vi "Main.vi"() -> ()   [LabVIEW 2016]
uses:
  type defs/action buttons.ctl
  type defs/mode buttons.ctl
  type defs/state.ctl
  type defs/data.ctl
  <vilib>/vision/Image Controls.llb/IMAQ Image.ctl
  <vilib>/myRIO/Instrument Drivers/Onboard IO/PWM/typedefs/PWM Reference.ctl
  <vilib>/myRIO/Common/Instrument Driver Framework/Utilities/typedefs/myRIO Generic Hardware Reference.ctl
  <vilib>/myRIO/Common/Instrument Driver Framework/Utilities/typedefs/Hardware Version Enum.ctl
  <vilib>/myRIO/Common/Instrument Driver Framework/Utilities/typedefs/myRIO v1.0 Reference.ctl
  <vilib>/myRIO/Common/Instrument Driver Framework/Utilities/typedefs/Generic FPGA Reference.ctl
  <vilib>/myRIO/Common/Instrument Driver Framework/myRIO v1.0/PWM/typedefs/PWM Channels Enum.ctl
  <vilib>/myRIO/Instrument Drivers/Onboard IO/PWM/typedefs/PWM Configuration.ctl
  <vilib>/userdefined/High Color/nirio_resource_hc.ctl
  <vilib>/myRIO/Instrument Drivers/Onboard IO/DIO/typedefs/DIO Reference.ctl
  <vilib>/myRIO/Common/Instrument Driver Framework/myRIO v1.0/DIO/typedefs/DIO Channels List.ctl
  <vilib>/myRIO/Common/Instrument Driver Framework/myRIO v1.0/DIO/typedefs/DIO Channels Enum.ctl
  <vilib>/myRIO/Common/Instrument Driver Framework/myRIO v1.0/Encoder/typedefs/Encoder Signal Mode.ctl
  <vilib>/myRIO/Instrument Drivers/Onboard IO/Encoder/typedefs/Encoder Reference.ctl
  <vilib>/myRIO/Common/Instrument Driver Framework/myRIO v1.0/Encoder/typedefs/Encoder Channels Enum.ctl
  <vilib>/myRIO/Common/Instrument Driver Framework/myRIO v1.0/Encoder/typedefs/Encoder Configuration v1.0.ctl
  type defs/task.ctl
  <vilib>/myRIO/Common/Instrument Driver Framework/Utilities/vis/Is FPGA Ref Available.vi
  <vilib>/myRIO/Common/Instrument Driver Framework/myRIO v1.0/PWM/vis/myRIO v1.1 Open PWM.vi
  <vilib>/myRIO/Instrument Drivers/Onboard IO/PWM/vis/Set Duty Cycle and Frequency.vi
  <vilib>/myRIO/Common/Instrument Driver Framework/myRIO v1.0/DIO/vis/myRIO v1.1 Open DIO.vi
  <vilib>/myRIO/Instrument Drivers/Onboard IO/DIO/vis/Write.vi
  <vilib>/myRIO/Common/Instrument Driver Framework/myRIO v1.0/Encoder/vis/myRIO v1.1 Open Encoder.vi
  <vilib>/myRIO/Instrument Drivers/Onboard IO/Encoder/vis/Read.vi
  <vilib>/myRIO/Instrument Drivers/Onboard IO/DIO/vis/Read.vi
  <vilib>/myRIO/Common/Instrument Driver Framework/Utilities/vis/Validate Channels.vi
  <vilib>/myRIO/Common/Instrument Driver Framework/myRIO v1.0/PWM/vis/myRIO v1.0 Reserve PWM.vi
  <vilib>/myRIO/Common/Instrument Driver Framework/myRIO v1.0/DIO/vis/myRIO v1.0 Reserve DIO.vi
  <vilib>/myRIO/Common/Instrument Driver Framework/myRIO v1.0/Encoder/vis/myRIO v1.0 Reserve Encoder.vi
  <vilib>/myRIO/Common/Instrument Driver Framework/myRIO v1.0/PWM/vis/myRIO v1.0 Build MUX Configuration PWM.vi
  <vilib>/myRIO/Common/Instrument Driver Framework/myRIO v1.0/Resource Manager/vis/myRIO v1.0 Reserve Channel List.vi
  <vilib>/myRIO/Common/Instrument Driver Framework/myRIO v1.0/DIO/vis/myRIO v1.0 Build MUX Configuration DIO.vi
  <vilib>/myRIO/Common/Instrument Driver Framework/myRIO v1.0/Encoder/vis/myRIO v1.0 Build MUX Configuration Encoder.vi
  <vilib>/myRIO/Common/Instrument Driver Framework/myRIO v1.0/Resource Manager/vis/myRIO v1.0 Create Configuration List.vi
  <vilib>/myRIO/Common/Instrument Driver Framework/myRIO v1.0/Resource Manager/vis/myRIO v1.0 Reserve Channel.vi
  <vilib>/myRIO/Common/Instrument Driver Framework/myRIO v1.0/Resource Manager/vis/myRIO v1.0 Unreserve Channel.vi
  <vilib>/myRIO/Common/Instrument Driver Framework/myRIO v1.0/Resource Manager/vis/myRIO v1.0 Build Mutex Name.vi
  <vilib>/Utility/VariantDataType/GetNumericInfo.vi
  <vilib>/Utility/error.llb/Error Cluster From Error Code.vi
  <vilib>/myRIO/Common/Instrument Driver Framework/myRIO v1.0/myRIO v1.1 Open.vi
  <vilib>/myRIO/Common/Instrument Driver Framework/Utilities/vis/IO Manager.vi
  <vilib>/myRIO/Common/Instrument Driver Framework/Utilities/vis/Configuration Manager.vi
  <vilib>/myRIO/Common/Instrument Driver Framework/myRIO v1.0/Resource Manager/vis/myRIO v1.0 Configure IO.vi
  <vilib>/myRIO/Common/Instrument Driver Framework/myRIO v1.0/myRIO v1.0 Close.vi
  <vilib>/myRIO/Common/Instrument Driver Framework/myRIO v1.0/PWM/vis/myRIO v1.0 Write PWM.vi
  <vilib>/myRIO/Common/Instrument Driver Framework/myRIO v1.0/DIO/vis/myRIO v1.0 Write DIO.vi
  <vilib>/myRIO/Common/Instrument Driver Framework/myRIO v1.0/Encoder/vis/myRIO v1.0 Configure Encoder.vi
  <vilib>/myRIO/Common/Instrument Driver Framework/myRIO v1.0/Encoder/vis/myRIO v1.0 Read Encoder.vi
  <vilib>/myRIO/Common/Instrument Driver Framework/myRIO v1.0/DIO/vis/myRIO v1.0 Read DIO.vi
  <vilib>/myRIO/Express VI/Onboard IO/PWM/PWM Express VI.xnode
  <vilib>/myRIO/Instrument Drivers/Onboard IO/PWM/vis/myRIO PWM Open.xnode
  <vilib>/myRIO/Express VI/Onboard IO/DO/DO Express VI.xnode
  <vilib>/myRIO/Instrument Drivers/Onboard IO/DIO/vis/myRIO DIO Open.xnode
  <vilib>/myRIO/Express VI/Onboard IO/Encoder/Encoder Express VI.xnode
  <vilib>/myRIO/Instrument Drivers/Onboard IO/Encoder/vis/myRIO Encoder Open.xnode
  <vilib>/myRIO/Common/Instrument Driver Framework/myRIO v1.0/Encoder/typedefs/Encoder Count Direction Enum.ctl
  <vilib>/myRIO/Express VI/Onboard Devices/LED/LED Express VI.xnode
  <vilib>/myRIO/Express VI/Onboard Devices/Button/Button Express VI.xnode
  <vilib>/vision/NI_Vision_Development_Module.lvlib
  <vilib>/myRIO/Instrument Drivers/Onboard IO/DIO/DIO.lvlib
  <vilib>/myRIO/Instrument Drivers/Onboard IO/PWM/PWM.lvlib
  <vilib>/myRIO/Instrument Drivers/Onboard IO/Encoder/Encoder.lvlib
panel:
  out "Pattern matches ball":bool
  out "Num of Matches (Color Pattern Matching 1)":i32
  out "Classes (Color Classification 1)":string[](array[string])
  out "Number of Matches (Pattern Matching 1)":i32
  out "Class (Particle Classification 1)":string
  out "Stopped":bool
  out "error out":errorcluster
  out "Boolean 2":bool
  in  "PWM 1":dbl(slide)=0.5 scale=0.0..1.0
  in  "PWM 2":dbl(slide)=0.5 scale=0.0..1.0
  out "take":bool
  in  "to give":bool
  out "Counter Value":i32
  out "Reset Counter":bool
  in  "Enum":enum16{"null", "one", "two", "stop"}(ring)=enum."two"
  out "back":bool
  out "number img":i32
  in  "mode buttons":T1
  out "image display":T2(plugin-control)
  in  "action buttons":T3
  in  "Stop":bool
  # "Machine\nVision\nApp"
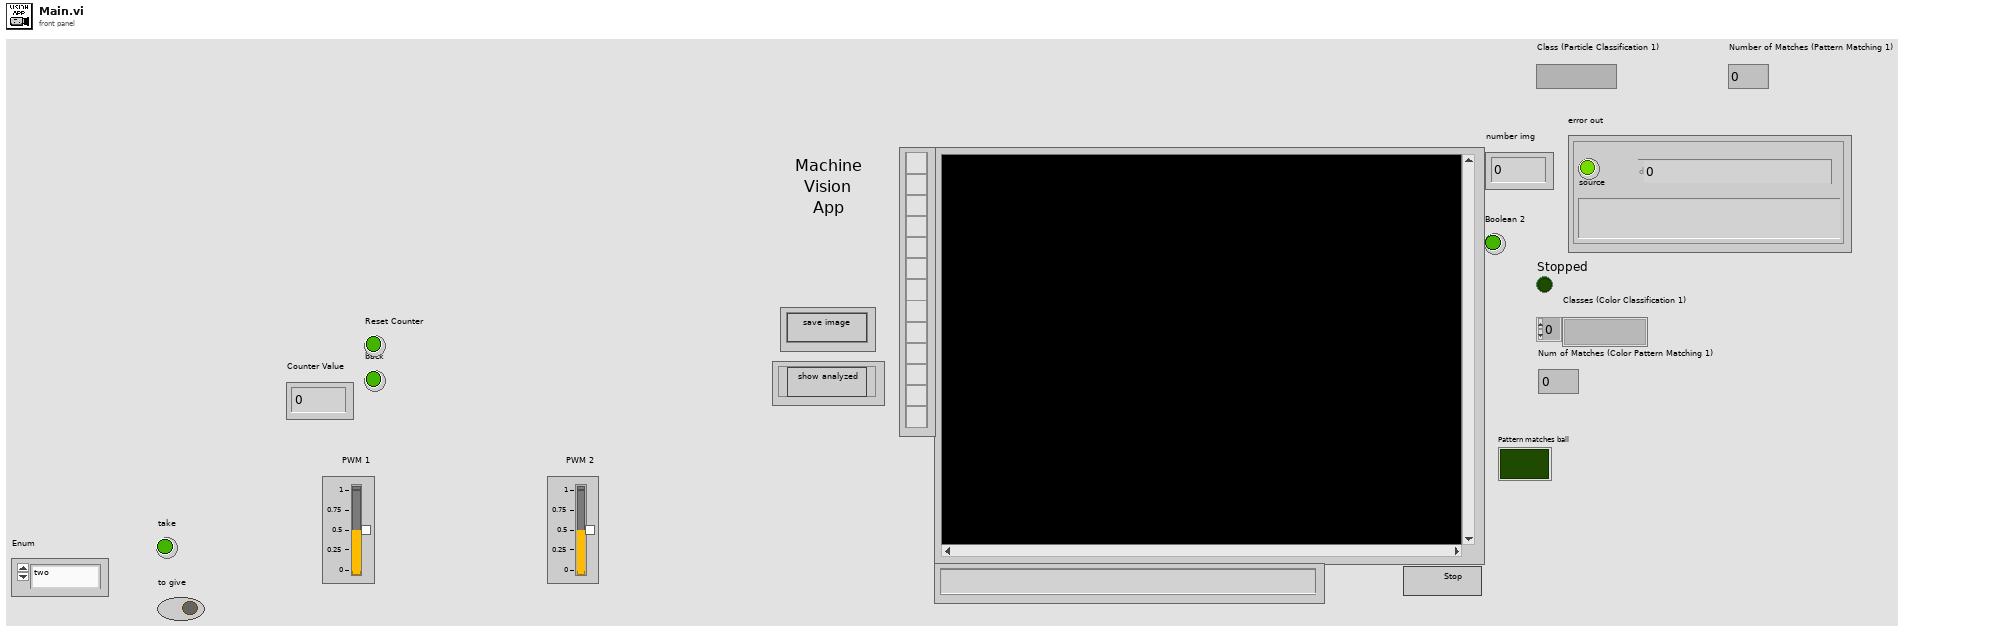
[diagram p1: front panel]
types:
  T1 = typedef "mode buttons.ctl" = cluster{"show analyzed":bool}
  T2 = typedef "IMAQ Image.ctl" = refnum<image>
  T3 = typedef "action buttons.ctl" = cluster{"save image":bool}
  T4 = typedef "data.ctl" = cluster{"save image":bool, "qsm":cluster{"Webcam image ref":T2, "Analyzed image ref":T2, "Stop webcam":bool}, " image ref":T2, "number img":i32}
  T5 = typedef "state.ctl" = enum16{"(qsm) schedule", "(qsm) initialize", "(qsm) release", "(qsm) clean up", "(qsm) shutdown", "(myRIO) initialize", "(myRIO) clean up", "(myRIO) update ports", "(image) get", "(image) analyze", "(image) overlay", "(image) show", "save image", "state A", "state B", "state C", "state D", "state E", "state F", "state G", "state H"}
  T6 = typedef "PWM.lvlib/PWM Reference.ctl" = cluster{"myRIO Reference":T7, "PWM Channels Enum":T11, "PWM Configuration":T12}
  T7 = typedef "myRIO Generic Hardware Reference.ctl" = cluster{"myRIO Model":T8, "myRIO Hardware Reference":T9}
  T8 = typedef "Hardware Version Enum.ctl" = enum16{"Unknown", "myRIO-1900", "myRIO-1950", "roboRIO", "NI ELVIS RIO CM"}
  T9 = typedef "myRIO v1.0 Reference.ctl" = cluster{"Generic FPGA Reference":T10, "Allow multiple opens":bool}
  T10 = typedef "Generic FPGA Reference.ctl" = refnum<k20>
  T11 = typedef "PWM Channels Enum.ctl" = enum16{"Not Connected", "C/PWM0", "C/PWM1", "A/PWM0", "A/PWM1", "A/PWM2", "B/PWM0", "B/PWM1", "B/PWM2", "PWM/PWM0", "PWM/PWM1", "PWM/PWM2", "PWM/PWM3", "PWM/PWM4", "PWM/PWM5", "PWM/PWM6", "PWM/PWM7", "PWM/PWM8", "PWM/PWM9"}
  T12 = typedef "PWM.lvlib/PWM Configuration.ctl" = cluster{"Frequency":dbl, "Duty Cycle":dbl}
  T13 = typedef "nirio_resource_hc.ctl" = tag
  T14 = typedef "Encoder.lvlib/Encoder Reference.ctl" = cluster{"myRIO Reference":T7, "Encoder Channels Enum":T15}
  T15 = typedef "Encoder Channels Enum.ctl" = enum16{"Not Connected", "C/ENC0", "C/ENC1", "A/ENC", "B/ENC", "DIO/ENC0", "DIO/ENC1", "DIO/ENC2", "DIO/ENC3", "DIO/ENC4"}
  T16 = typedef "Encoder Signal Mode.ctl" = enum16{"Quadrature phase signal", "Step and direction signal"}
  T17 = typedef "DIO.lvlib/DIO Reference.ctl" = cluster{"myRIO Reference":T7, "DIO Channels List":T18}
  T18 = typedef "DIO Channels List.ctl" = T19[]
  T19 = typedef "DIO Channels Enum.ctl" = enum16{"Not Connected", "C/DIO0", "C/DIO1", "C/DIO2", "C/DIO3", "C/DIO4", "C/DIO5", "C/DIO6", "C/DIO7", "A/DIO0", "A/DIO1", "A/DIO2", "A/DIO3", "A/DIO4", "A/DIO5", "A/DIO6", "A/DIO7", "A/DIO8", "A/DIO9", "A/DIO10", "A/DIO11", "A/DIO12", "A/DIO13", "A/DIO14", "A/DIO15", "B/DIO0", "B/DIO1", "B/DIO2", "B/DIO3", "B/DIO4", "B/DIO5", "B/DIO6", "B/DIO7", "B/DIO8", "B/DIO9", "B/DIO10", "B/DIO11", "B/DIO12", "B/DIO13", "B/DIO14", "B/DIO15", "LED0", "LED1", "LED2", "LED3", "Button0", "DIO/DIO0", "DIO/DIO1", "DIO/DIO2", "DIO/DIO3", "DIO/DIO4", "DIO/DIO5", "DIO/DIO6", "DIO/DIO7", "DIO/DIO8", "DIO/DIO9", "SPI/CS0", "SPI/CS1", "SPI/CS2", "SPI/CS3", "LED RADIO (Green)", "LED RADIO (Red)", "LED COMM (Green)", "LED COMM (Red)", "LED MODE (Green)", "LED MODE (Red)"}
  T20 = typedef "task.ctl" = T5[]
  T21 = typedef "Image Type" = u32
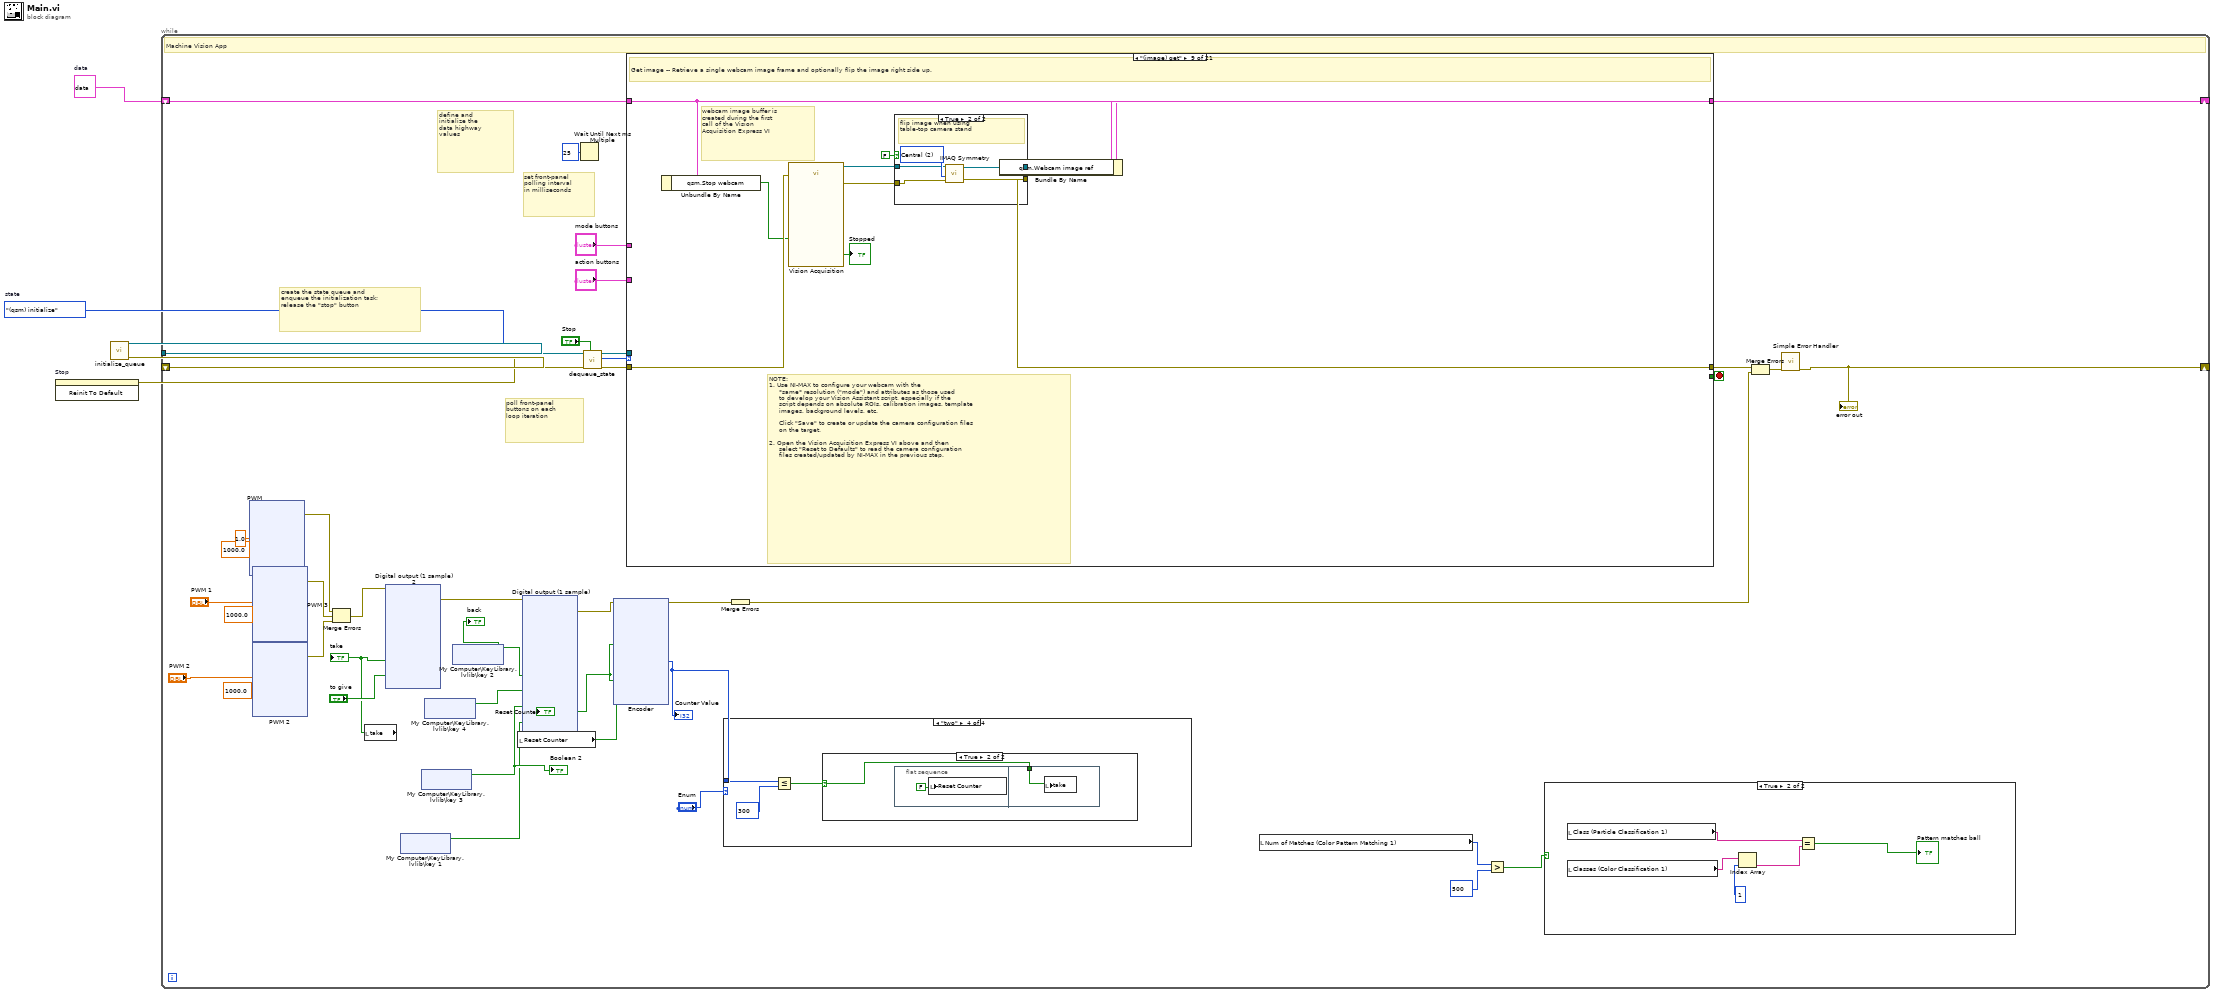
[diagram p0: block diagram]
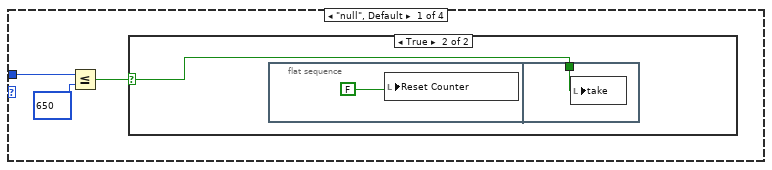
[diagram p3: hidden frame]
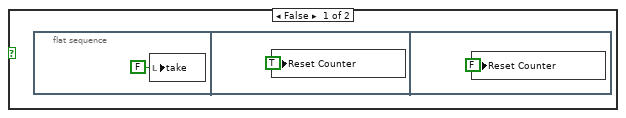
[diagram p4: hidden frame]
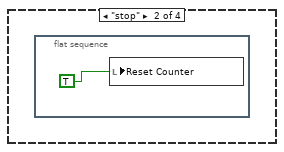
[diagram p5: hidden frame]
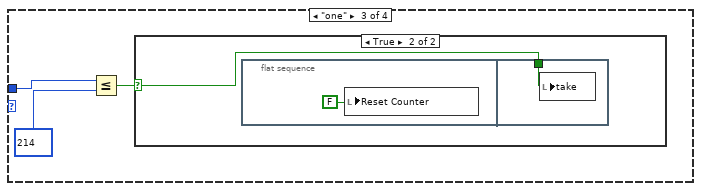
[diagram p6: hidden frame]
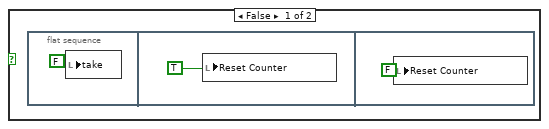
[diagram p7: hidden frame]
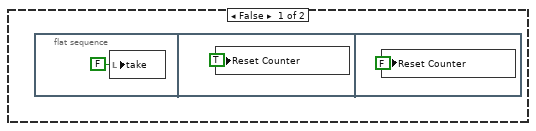
[diagram p8: hidden frame]
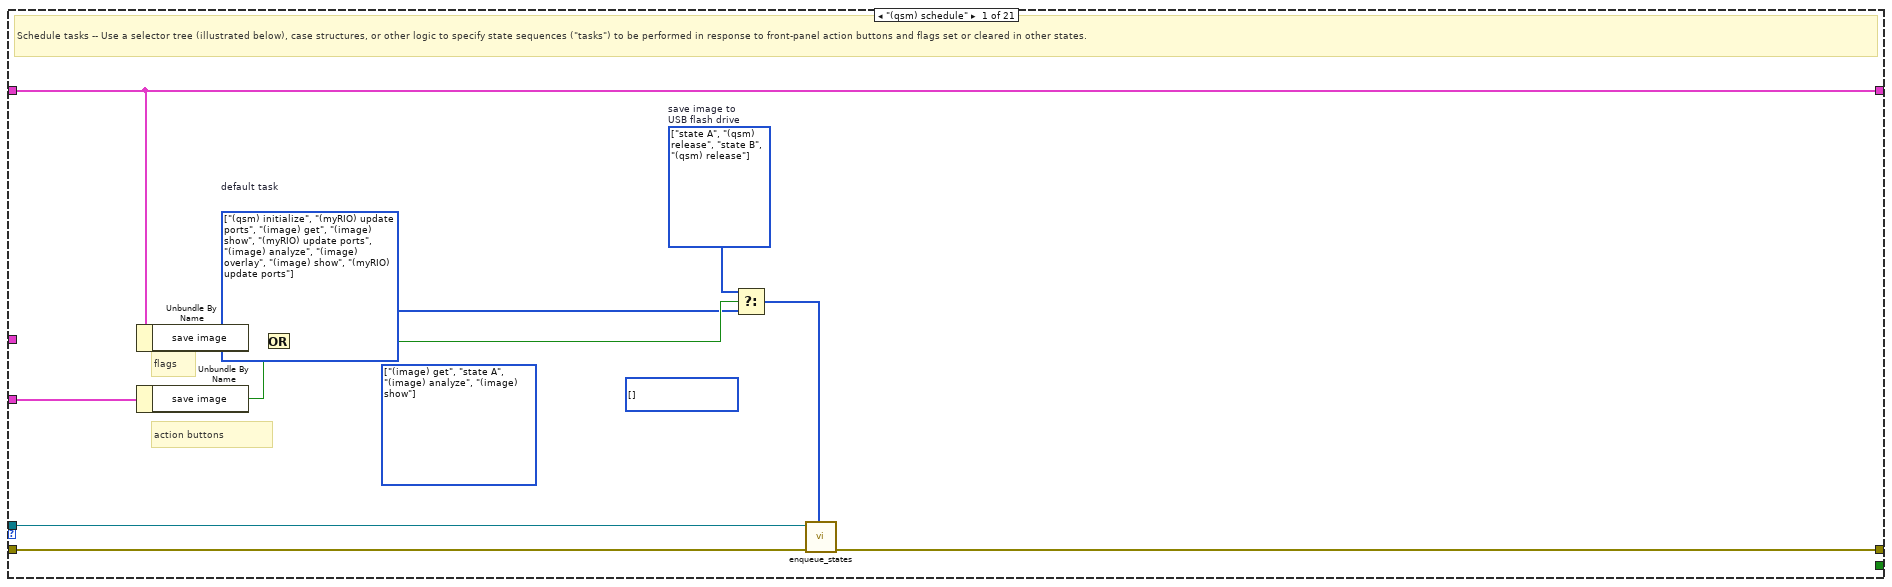
[diagram p9: hidden frame]
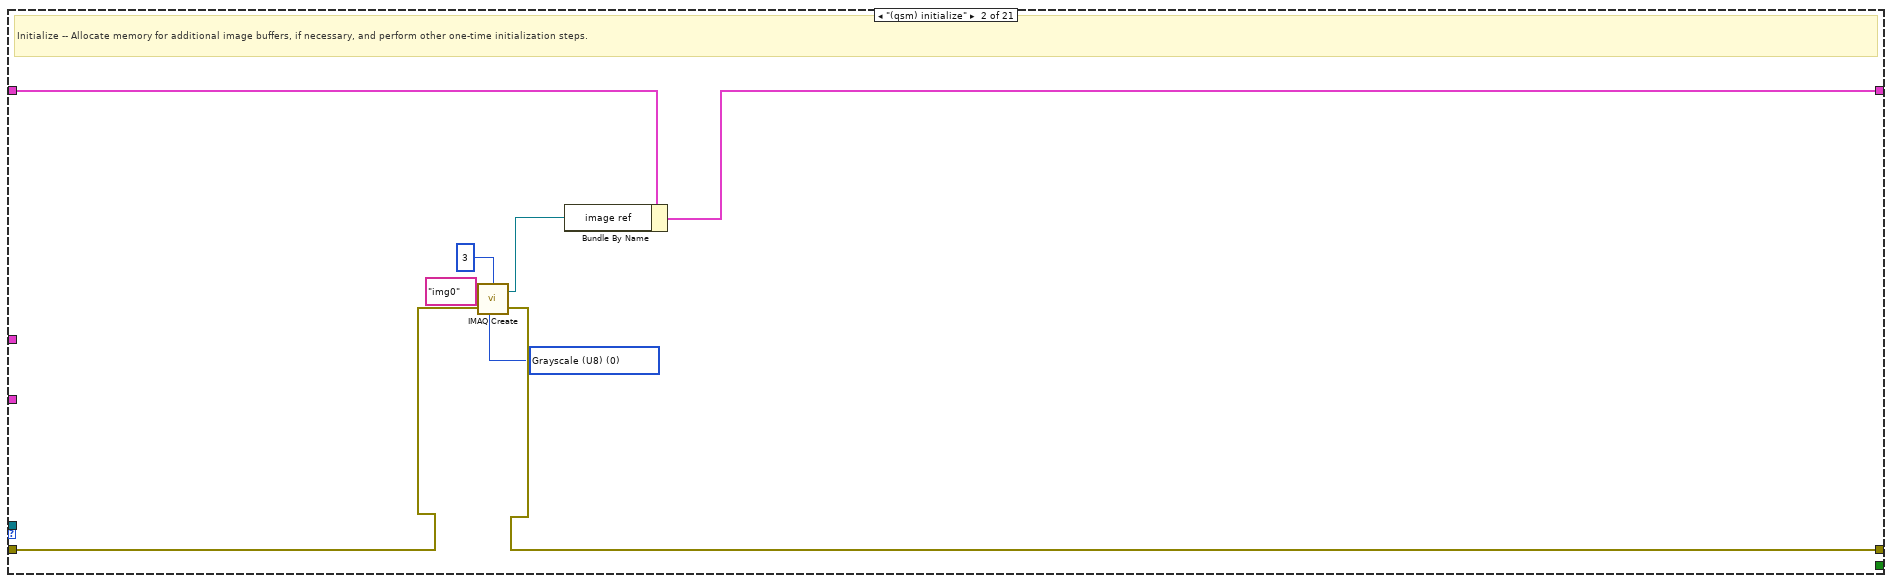
[diagram p10: hidden frame]
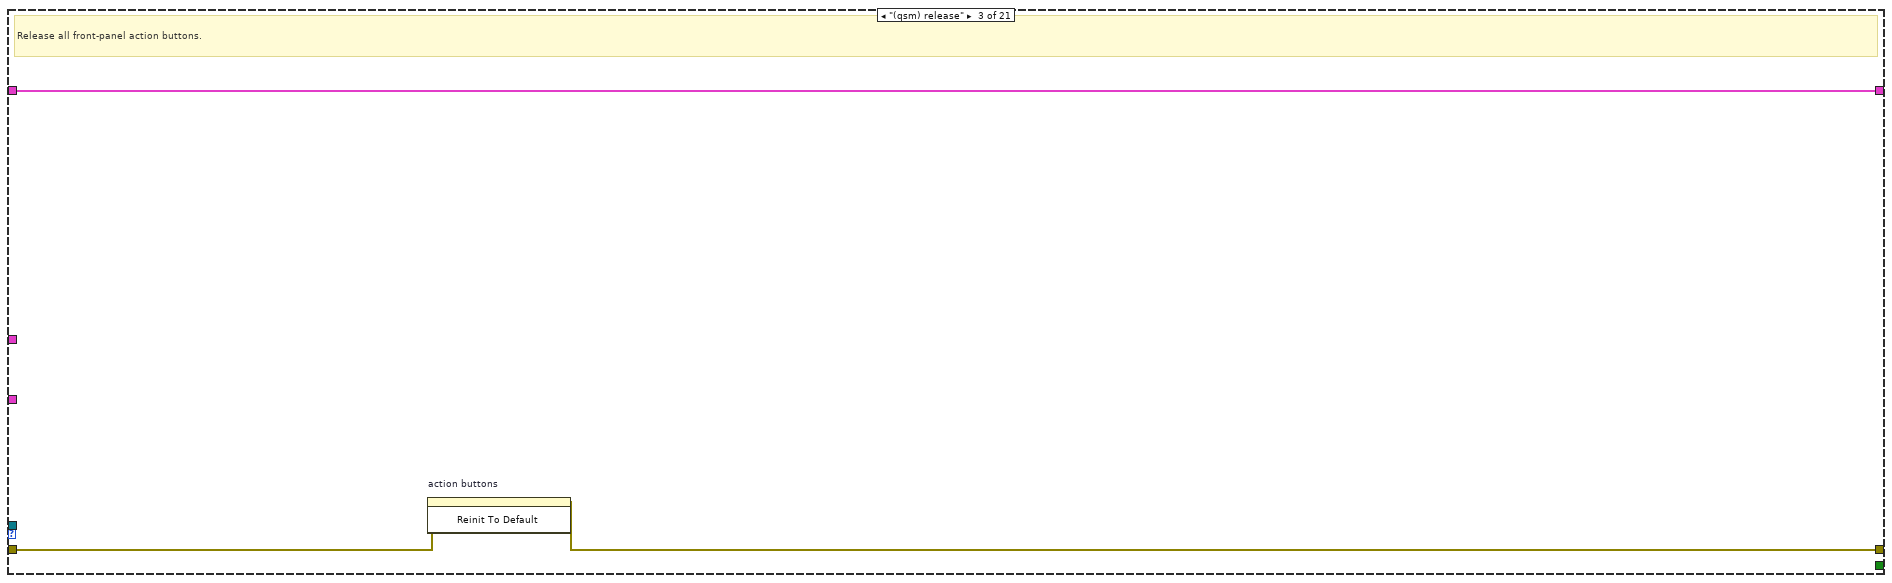
[diagram p11: hidden frame]
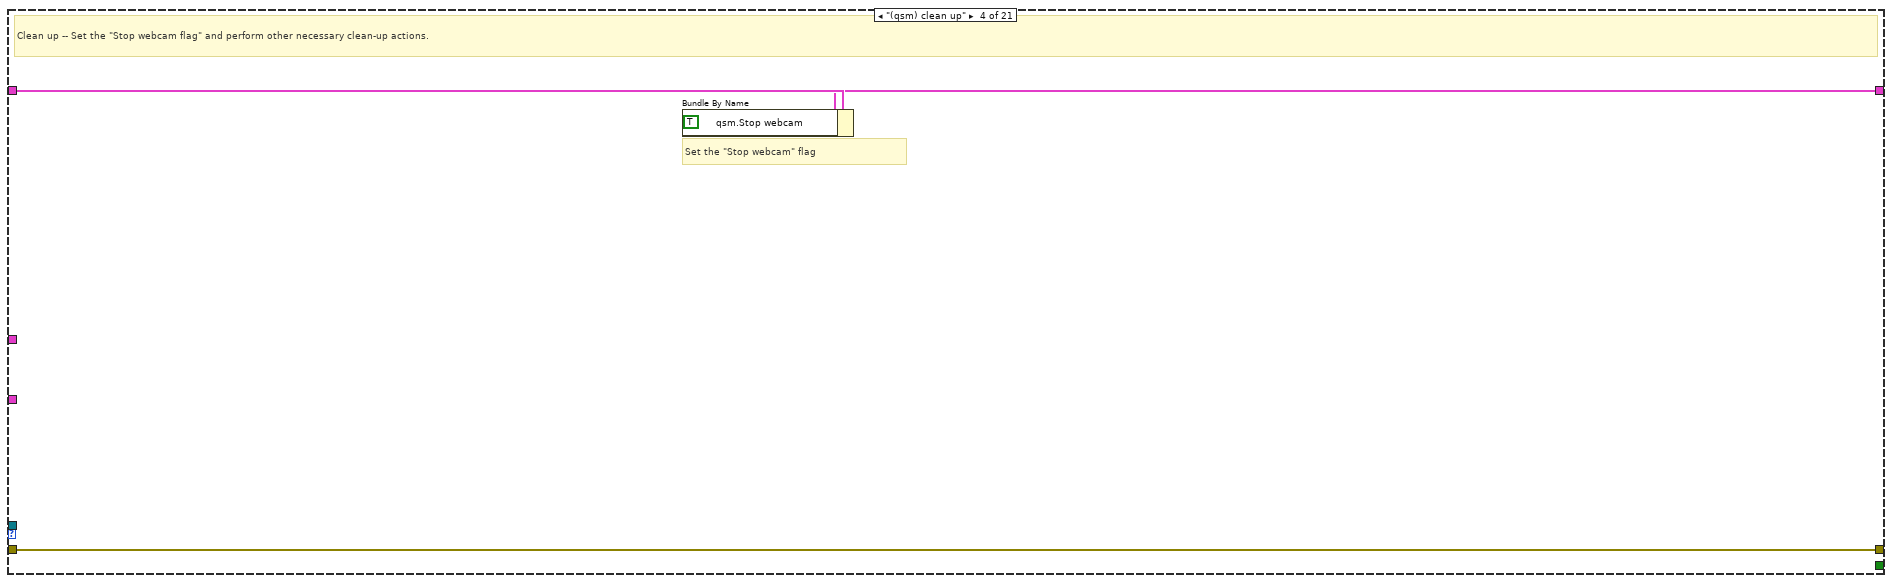
[diagram p12: hidden frame]
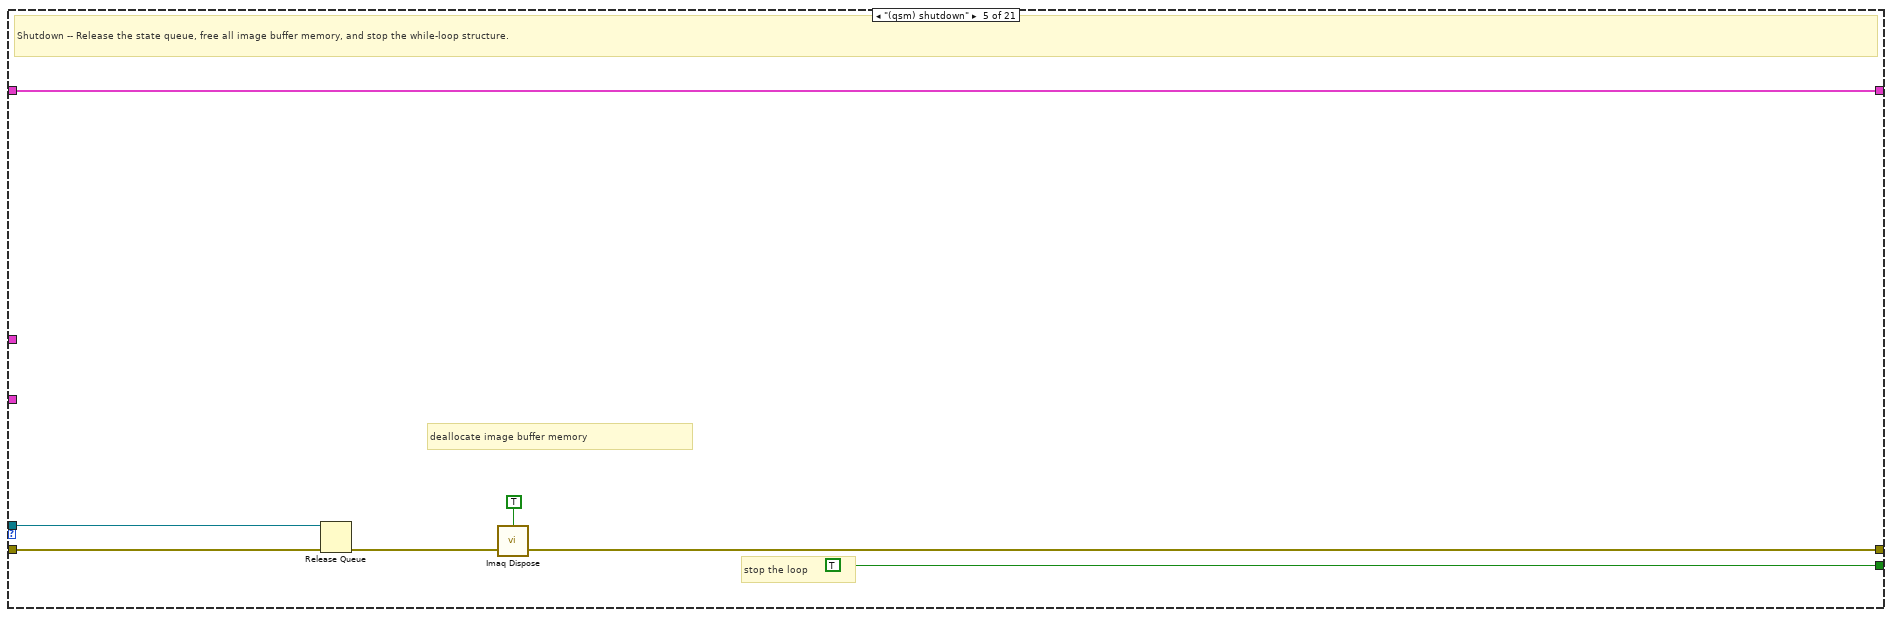
[diagram p13: hidden frame]
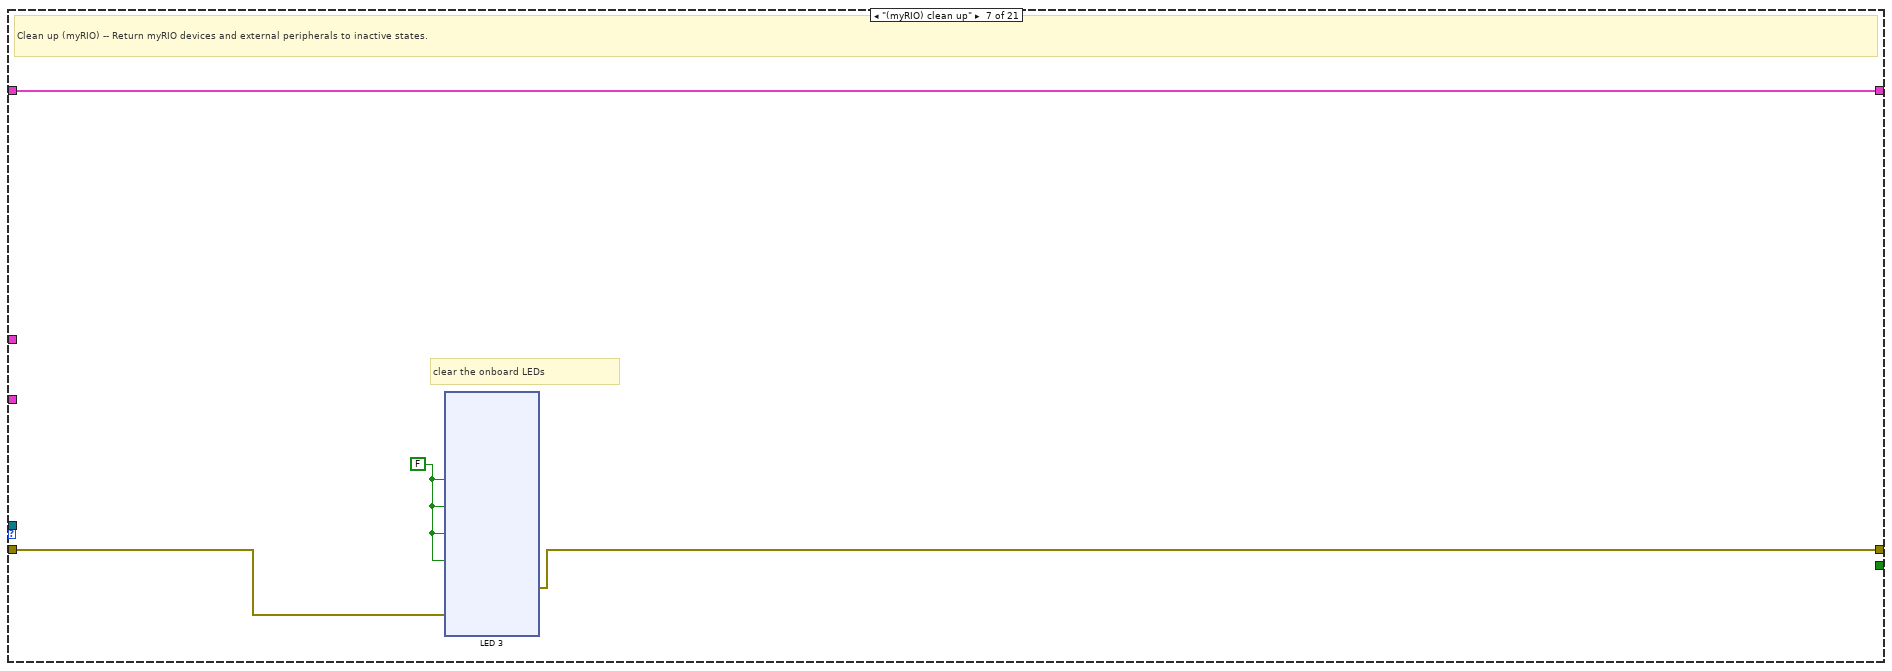
[diagram p15: hidden frame]
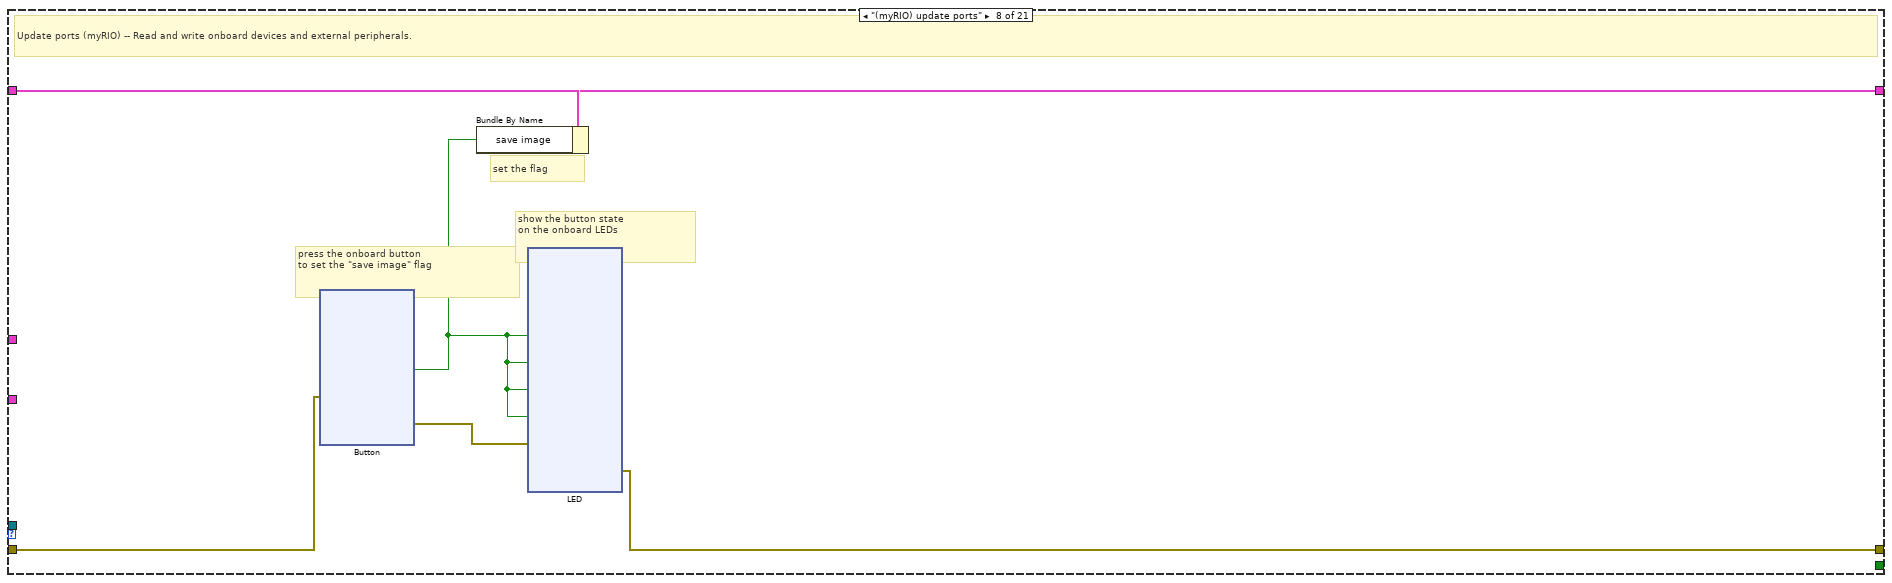
[diagram p16: hidden frame]
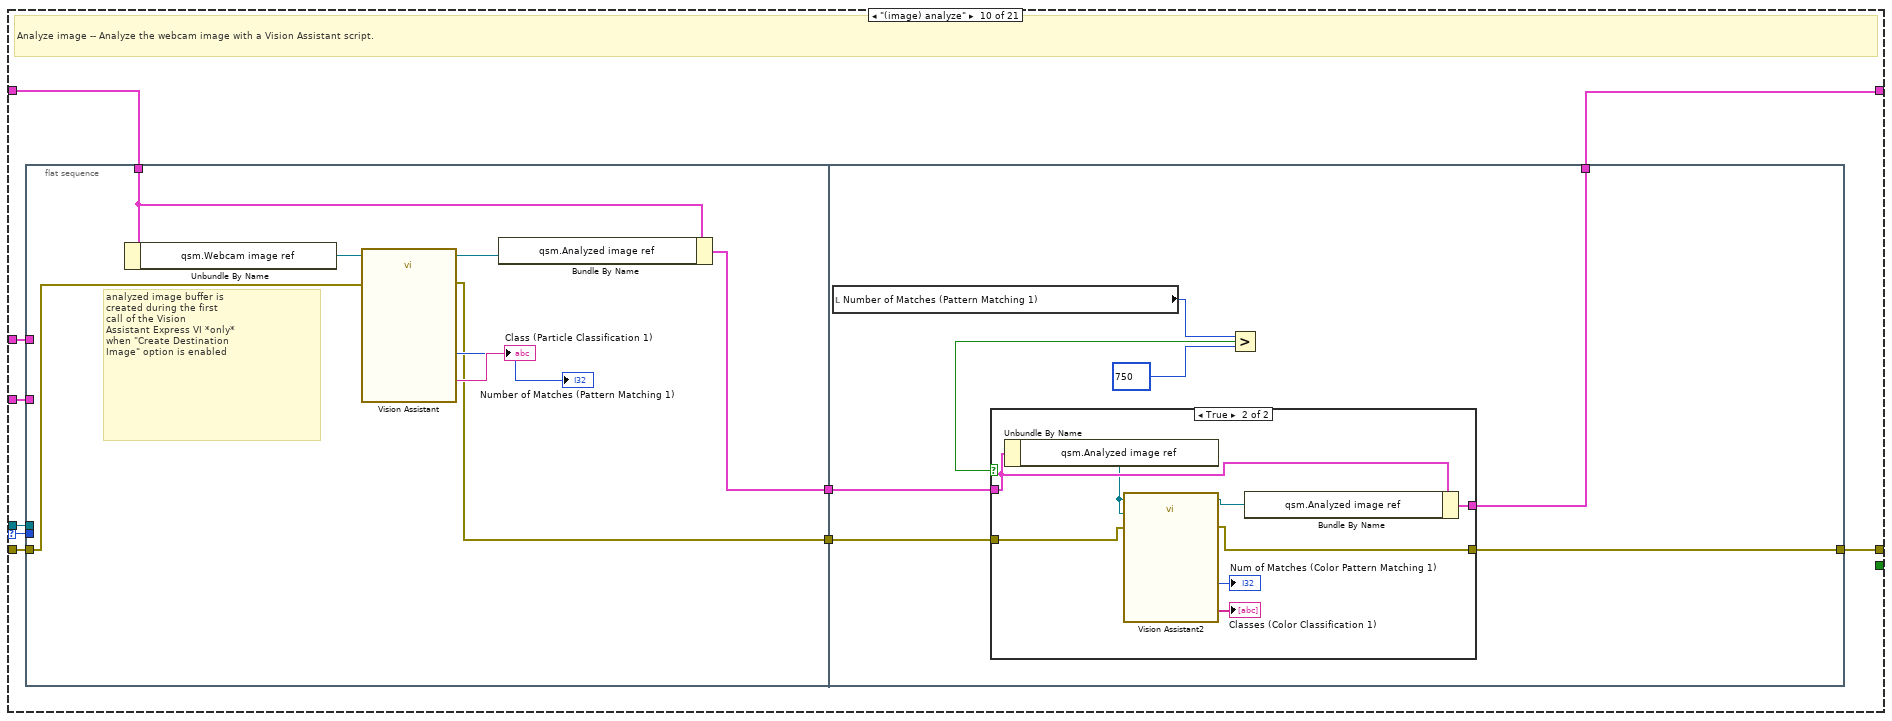
[diagram p18: hidden frame]
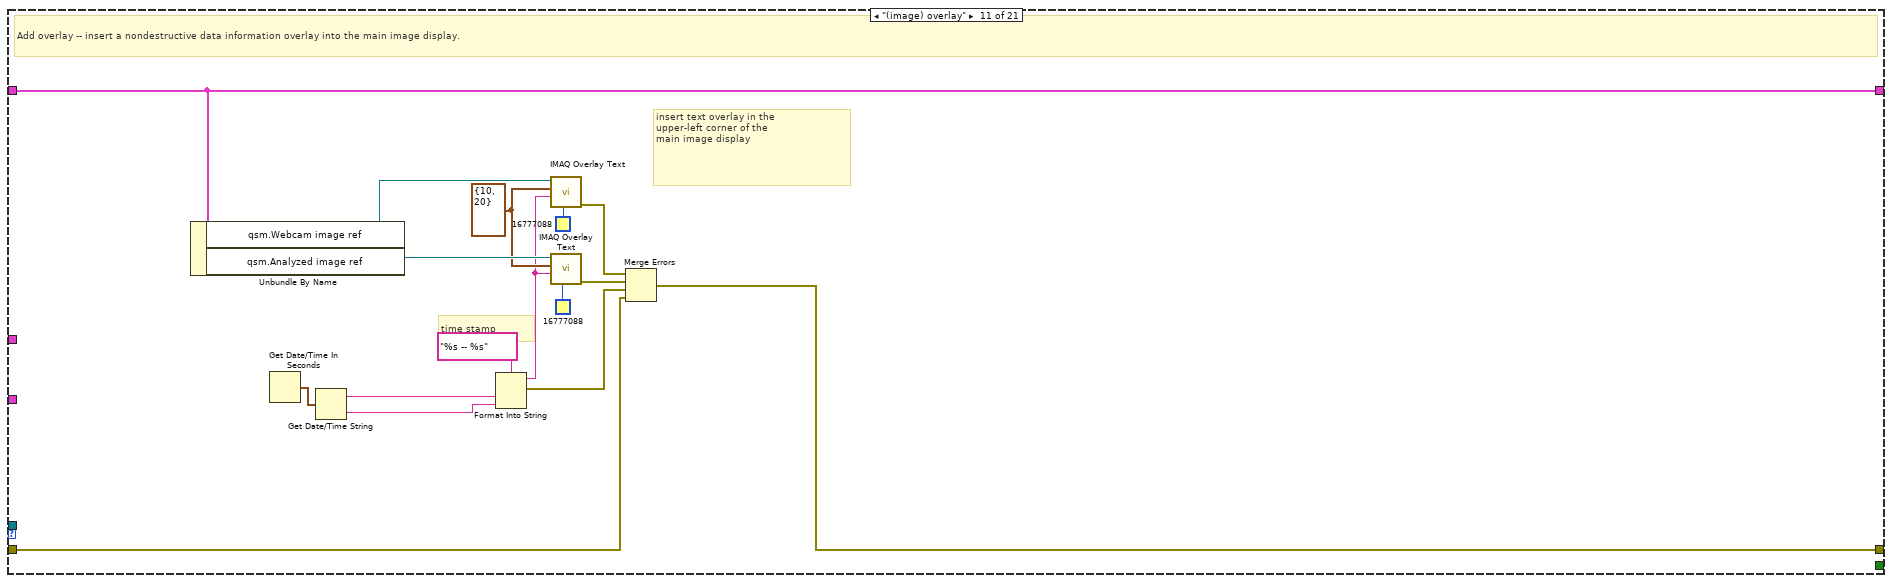
[diagram p20: hidden frame]
diagram:
  w5 = T4 {"save image"=FALSE, "qsm"={"Webcam image ref"=refnum, "Analyzed image ref"=refnum, "Stop webcam"=FALSE}, " image ref"=refnum, "number img"=0}  # data
  w1 = state."(qsm) initialize"  # state
  n1 = invoke on="Stop" class="Bool" method="Reinit To Default"() -> (error out=w2:errorcluster)  [unwired: 3 in, 2 out]
  n2 = call "initialize_queue.vi"("error in (no error)"=w2, "state"=w1) -> ("error out"=w4:errorcluster, "queue out"=w3:refnum<queue>)  [unwired: 8 in]
  n3 = while {
    shift-right: [w14] -> _
    shift-left: w4 -> [w38]
    tunnel: w3 -> [w39]
    shift-right: [w42] -> _
    shift-left: w5 -> [w43]
    stop <- w41 stop-if-true
    # "define and \ninitialize the \ndata highway\nvalues"
    # "create the state queue and\nenqueue the initialization task;\nrelease the \"stop\" button"
    # "set front-panel\npolling interval\nin milliseconds"
    # "poll front-panel\nbuttons on each\nloop iteration"
    # "Machine Vision App"
    n4 = xnode "PWM"("Duty Cycle"=1.0, "Frequency [Hz]"=1000.0) -> ("error out"=w18:errorcluster)  [unwired: 1 in]
    n5 = xnode "PWM 3"("Duty Cycle"="PWM 1", "Frequency [Hz]"=1000.0) -> ("error out"=w32:errorcluster)  [unwired: 1 in]
    n6 = xnode "PWM 2"("Duty Cycle"="PWM 2", "Frequency [Hz]"=1000.0) -> ("error out"=w31:errorcluster)  [unwired: 1 in]
    n7 = Merge Errors(w18, w32, w31) -> (w26:errorcluster)
    n8 = local read "take"() -> (w21:bool)
    "take" <- w21
    n9 = xnode "Digital output (1 sample) 2"("B/DIO5 (Pin 21)"=w21, "B/DIO6 (Pin 23)"="to give", "error in (no error)"=w26) -> ("error out"=w15:errorcluster)
    n10 = shared-variable "My Computer\\KeyLibrary.lvlib\\key 1"() -> (w9:bool)  [unwired: 1 in, 1 out]
    n11 = shared-variable "My Computer\\KeyLibrary.lvlib\\key 3"() -> (w11:bool)  [unwired: 1 in, 1 out]
    "Boolean 2" <- w11
    n12 = shared-variable "My Computer\\KeyLibrary.lvlib\\key 4"() -> (w10:bool)  [unwired: 1 in, 1 out]
    n13 = shared-variable "My Computer\\KeyLibrary.lvlib\\key 2"() -> (w12:bool)  [unwired: 1 in, 1 out]
    "back" <- w12
    n14 = local read "Reset Counter"() -> (w20:bool)
    "Reset Counter" <- w20
    n15 = xnode "Digital output (1 sample)"("A/DIO5 (Pin 21)"=w12, "A/DIO6 (Pin 23)"=w10, "A/DIO7 (Pin 25)"=w11, "A/DIO13 (Pin 26)"=w9, "error in (no error)"=w15) -> ("error out"=w24:errorcluster)
    n16 = Wait Until Next ms Multiple(millisecond multiple=u32 25) -> ()  [unwired: 1 out]
    n17 = call "dequeue_state.vi"("stop"="Stop", "error in (no error)"=w38, "queue in"=w39) -> ("error out"=w40:errorcluster, "state"=w33:T5, "queue out"=w36:refnum<queue>)  [unwired: 6 in]
    n18 = xnode "Encoder"("Reset Counter"=w20, "error in (no error)"=w24) -> ("Counter Value"=w22:i32, "error out"=w23:errorcluster)  [unwired: 2 out]
    "Counter Value" <- w22
    n19 = case shown="\"(image) get\"" w33 {
      selector: w33 -> [_ _ _ _ _ _ _ _ _ w478 _ _ _ _ _ _ _ _ _ _ _]
      tunnel: w40 -> [w310 w322 w324 w326 w335 w337 w340 w384 w469 w477 w512 w530 w538 w562 w605 w649 w651 w653 w654 w656 w659]
      tunnel: w36 -> [w311 _ _ _ w334 _ _ _ _ w479 _ _ _ _ _ _ _ _ _ _ _]
      tunnel: [w312 w321 w323 w326 w330 w337 w339 w382 w464 w482 w521 w530 w539 w559 w606 w649 w651 w653 w654 w656 w659] -> w45
      tunnel: "action buttons" -> [w314 _ _ _ _ _ _ _ _ w480 _ _ _ _ _ _ _ _ _ _ _]
      tunnel: w43 -> [w313 w316 w325 w328 w333 w338 w342 w386 w462 w486 w513 w531 w543 w563 w604 w648 w650 w652 w655 w657 w658]
      tunnel: [w313 w315 w325 w327 w333 w338 w342 w385 w468 w485 w513 w531 w542 w563 w602 w648 w650 w652 w655 w657 w658] -> w42
      tunnel: [_ _ _ _ TRUE _ _ _ _ _ _ _ _ _ _ _ _ _ _ _ _] -> w41
      tunnel: "mode buttons" -> [_ _ _ _ _ _ _ _ _ w481 _ w529 w540 _ _ _ _ _ _ _ _]
      frame "(qsm) schedule" {
        (unwired) T20 [enum."(image) get", enum."state A", enum."(image) analyze", enum."(image) show"] items=["(qsm) schedule", "(qsm) initialize", "(qsm) release", "(qsm) clean up", "(qsm) shutdown", "(myRIO) initialize", "(myRIO) clean up", "(myRIO) update ports", "(image) get", "(image) analyze", "(image) overlay", "(image) show", "save image", "state A", "state B", "state C", "state D", "state E", "state F", "state G", "state H"] ("task")
        (unwired) T5[] [] items=["(qsm) schedule", "(qsm) initialize", "(qsm) release", "(qsm) clean up", "(qsm) shutdown", "(myRIO) initialize", "(myRIO) clean up", "(myRIO) update ports", "(image) get", "(image) analyze", "(image) overlay", "(image) show", "save image", "state A", "state B", "state C", "state D", "state E", "state F", "state G", "state H"]
        w306 = T20 [enum."state A", enum."(qsm) release", enum."state B", enum."(qsm) release"] items=["(qsm) schedule", "(qsm) initialize", "(qsm) release", "(qsm) clean up", "(qsm) shutdown", "(myRIO) initialize", "(myRIO) clean up", "(myRIO) update ports", "(image) get", "(image) analyze", "(image) overlay", "(image) show", "save image", "state A", "state B", "state C", "state D", "state E", "state F", "state G", "state H"]  # save image to USB flash drive
        w304 = T20 [enum."(qsm) initialize", enum."(myRIO) update ports", enum."(image) get", enum."(image) show", enum."(myRIO) update ports", enum."(image) analyze", enum."(image) overlay", enum."(image) show", enum."(myRIO) update ports"] items=["(qsm) schedule", "(qsm) initialize", "(qsm) release", "(qsm) clean up", "(qsm) shutdown", "(myRIO) initialize", "(myRIO) clean up", "(myRIO) update ports", "(image) get", "(image) analyze", "(image) overlay", "(image) show", "save image", "state A", "state B", "state C", "state D", "state E", "state F", "state G", "state H"]  # default task
        # "action buttons"
        # "flags"
        # "Schedule tasks -- Use a selector tree (illustrated below), case structures, or other logic to specify state sequences (\"tasks\") to be performed in response to front-panel action buttons and flags set or cleared in other states."
        n20 = Unbundle By Name "Unbundle By Name"(w313) -> ("save image"=w309:bool)
        n21 = Unbundle By Name(w314) -> ("save image"=w308:bool)
        n22 = Or(x=w309, y=w308) -> (x .or. y?=w307:bool)
        n23 = Select(t=w306, s=w307, f=w304) -> (s? t:f=w305:T20)
        n24 = call "enqueue_states.vi"("task"=w305, "error in"=w310, "queue in"=w311) -> ("error out"=w312:errorcluster)  [unwired: 6 in, 1 out]
      }
      frame "(qsm) initialize" {
        w319 = T21 0 items=["Grayscale (U8)", "Grayscale (I16)", "Grayscale (SGL)", "Complex (CSG)", "RGB (U32)", "HSL (U32)", "RGB (U64)", "Grayscale (U16)"] ("Image Type")
        # "Initialize -- Allocate memory for additional image buffers, if necessary, and perform other one-time initialization steps."
        n25 = call "IMAQ Create"("Border Size"=3, "Image Name"="img0", "Image Type"=w319, "error in (no error)"=w322) -> ("New Image"=w317:T2, "error out"=w321:errorcluster)  [unwired: 1 in]
        n26 = Bundle By Name(cluster=w316, "image ref"=w317) -> (w315:T4)
      }
      frame "(qsm) release" {
        # "Release all front-panel action buttons."
        n27 = invoke on="action buttons" class="Clust (strict)" method="Reinit To Default"(error in=w324) -> (error out=w323:errorcluster)  [unwired: 2 in, 2 out]
      }
      frame "(qsm) clean up" {
        # "Set the \"Stop webcam\" flag"
        # "Clean up -- Set the \"Stop webcam flag\" and perform other necessary clean-up actions."
        n28 = Bundle By Name(cluster=w328, "qsm.Stop webcam"=TRUE) -> (w327:T4)
      }
      frame "(qsm) shutdown" {
        # "deallocate image buffer memory"
        # "stop the loop"
        # "Shutdown -- Release the state queue, free all image buffer memory, and stop the while-loop structure."
        n29 = Release Queue(queue=w334, error in (no error)=w335) -> (error out=w331:errorcluster)  [unwired: 1 in, 2 out]
        n30 = call "Imaq Dispose"("All Images? (No)"=TRUE, "error in (no error)"=w331) -> ("error out"=w330:errorcluster)  [unwired: 4 in]
      }
      frame "(myRIO) initialize" {
        # "Initialize (myRIO) -- Open channels, configure devices, send setup strings to peripherals, etc."
      }
      frame "(myRIO) clean up" {
        w341 = FALSE ("LED3")
        # "clear the onboard LEDs"
        # "Clean up (myRIO) -- Return myRIO devices and external peripherals to inactive states."
        n31 = xnode "LED 3"("LED0"=w341, "LED1"=w341, "LED2"=w341, "LED3"=w341, "error in (no error)"=w340) -> ("error out"=w339:errorcluster)
      }
      frame "(myRIO) update ports" {
        # "show the button state\non the onboard LEDs"
        # "set the flag"
        # "press the onboard button\nto set the \"save image\" flag"
        # "Update ports (myRIO) -- Read and write onboard devices and external peripherals."
        n32 = xnode "Button"("error in (no error)"=w384) -> ("Value"=w381:bool, "error out"=w383:errorcluster)
        n33 = Bundle By Name "Bundle By Name"(cluster=w386, "save image"=w381) -> (w385:T4)
        n34 = xnode "LED"("LED0"=w381, "LED1"=w381, "LED2"=w381, "LED3"=w381, "error in (no error)"=w383) -> ("error out"=w382:errorcluster)
      }
      frame "(image) get" {
        # "webcam image buffer is\ncreated during the first\ncall of the Vision\nAcquisition Express VI"
        # "NOTE:\n1. Use NI-MAX to configure your webcam with the\n     *same* resolution (\"mode\") and attributes as those used \n     to develop your Vision Assistant script, especially if the\n     script depends on absolute ROIs, calibration images, template\n     images, background levels, etc.\n \n     Click \"Save\" to create or update the camera configuration files\n     on the target.\n\n2. Open the Vision Acquisition Express VI above and then\n     select \"Reset to Defaults\" to read the camera configuration\n     files created/updated by NI-MAX in the previous step."
        # "Get image -- Retrieve a single webcam image frame and optionally flip the image right side up."
        n35 = Unbundle By Name(w462) -> ("qsm.Stop webcam"=w461:bool)
        n36 = call "Vision Acquisition"("Stop (F)"=w461, "error in"=w469) -> ("Image Out"=w467:T2, "Stopped"=→"Stopped":bool, "error out"=w465:errorcluster)  [unwired: 22 in, 1 out]
        n37 = case shown="True" FALSE {
          tunnel: w467 -> [w471 w475]
          tunnel: [w471 w474] -> w466
          tunnel: w465 -> [w470 w473]
          tunnel: [w470 w472] -> w464
          frame False {
            # "use webcam image as-is"
          }
          frame True {
            w476 = u32 2 items=["Horizontal", "Vertical", "Central", "1st Diagonal", "2nd Diagonal"] ("Type of Symmetry")
            # "flip image when using\ntable-top camera stand"
            n38 = call "IMAQ Symmetry"("error in (no error)"=w473, "Type of Symmetry"=w476, "Image Src"=w475) -> ("error out"=w472:errorcluster, "Image Dst Out"=w474:T2)  [unwired: 2 in]
          }
        }
        n39 = Bundle By Name(cluster=w462, "qsm.Webcam image ref"=w466) -> (w468:T4)
      }
      frame "(image) analyze" {
        # "Analyze image -- Analyze the webcam image with a Vision Assistant script."
        n40 = flat-sequence {
          tunnel: w486 -> [w494]
          tunnel: [w489] -> w484
          tunnel: [w488] -> w483
          tunnel: w481 -> [_]
          tunnel: w480 -> [_]
          tunnel: w479 -> [_]
          tunnel: w478 -> [_]
          tunnel: w477 -> [w487]
          tunnel: [w497] -> w485
          tunnel: w484 -> [w498]
          tunnel: w483 -> [w496]
          tunnel: [w495] -> w482
          frame #0 {
            # "analyzed image buffer is\ncreated during the first\ncall of the Vision\nAssistant Express VI *only*\nwhen \"Create Destination\nImage\" option is enabled"
            n41 = Unbundle By Name "Unbundle By Name"(w494) -> ("qsm.Webcam image ref"=w493:T2)
            n42 = call "Vision Assistant"("Image In"=w493, "error in"=w487) -> ("Image Out"=w492:T2, "Class (Particle Classification 1)"=→"Class (Particle Classification 1)":string, "Number of Matches (Pattern Matching 1)"=→"Number of Matches (Pattern Matching 1)":i32, "error out"=w488:errorcluster)  [unwired: 22 in]
            n43 = Bundle By Name "Bundle By Name"(cluster=w494, "qsm.Analyzed image ref"=w492) -> (w489:T4)
          }
          frame #1 {
            n44 = local read "Number of Matches (Pattern Matching 1)"() -> (w501:i32)
            n45 = Greater?(x=w501, y=750) -> (0:w499:bool)
            n46 = case shown="True" w499 {
              tunnel: w498 -> [w503 w508]
              tunnel: [w503 w507] -> w497
              tunnel: w496 -> [w502 w506]
              tunnel: [w502 w505] -> w495
              frame False {
              }
              frame True {
                n47 = Unbundle By Name(w508) -> ("qsm.Analyzed image ref"=w504:T2)
                n48 = call "Vision Assistant2"("Image In"=w504, "Image Dst"=w504, "error in"=w506) -> ("Image Out"=w511:T2, "Classes (Color Classification 1)"=→"Classes (Color Classification 1)":string[], "Number of Matches (Color Pattern Matching 1)"=→"Num of Matches (Color Pattern Matching 1)":i32, "error out"=w505:errorcluster)  [unwired: 21 in]
                n49 = Bundle By Name(cluster=w508, "qsm.Analyzed image ref"=w511) -> (w507:T4)
              }
            }
          }
        }
      }
      frame "(image) overlay" {
        w523 = cluster{"X":i32, "Y":i32} {"X"=10, "Y"=20} ("Origin")
        # "time stamp"
        # "insert text overlay in the\nupper-left corner of the \nmain image display"
        # "Add overlay -- insert a nondestructive data information overlay into the main image display."
        n50 = Unbundle By Name "Unbundle By Name"(w513) -> ("qsm.Webcam image ref"=w524:T2, "qsm.Analyzed image ref"=w527:T2)
        n51 = Get Date/Time In Seconds() -> (seconds since 1Jan1904=w517:timestamp)
        n52 = Get Date/Time String(seconds (now)=w517) -> (date string=w516:string, time string=w515:string)  [unwired: 2 in]
        n53 = Format Into String "Format Into String"(format string="%s -- %s", w516, w515) -> (resulting string=w518:string, error out=w514:errorcluster)  [unwired: 2 in]
        n54 = call "IMAQ Overlay Text"("Text Color (black)"=u32 16777088, "String"=w518, "Origin"=w523, "Image"=w524) -> ("error out"=w520:errorcluster)  [unwired: 6 in, 1 out]
        n55 = call "IMAQ Overlay Text"("Text Color (black)"=u32 16777088, "String"=w518, "Origin"=w523, "Image"=w527) -> ("error out"=w522:errorcluster)  [unwired: 6 in, 1 out]
        n56 = Merge Errors "Merge Errors"(w520, w522, w514, w512) -> (w521:errorcluster)
      }
      frame "(image) show" {
        # "Show image -- Select from among the available image buffers to show on the main image display; use a selector tree or case structure."
        n57 = Unbundle By Name "Unbundle By Name"(w529) -> ("show analyzed"=w528:bool)
        n58 = Unbundle By Name "Unbundle By Name"(w531) -> ("qsm.Analyzed image ref"=w534:T2, "qsm.Webcam image ref"=w533:T2)
        n59 = Select(t=w534, s=w528, f=w533) -> (s? t:f=→"image display":T2)
      }
      frame "save image" {
        # "check for USB flash drive\nconnected to myRIO"
        # "clear the flag that was set by\npressing the myRIO onboard button"
        # "Save image (example of an application-specific state) -- Save either the original webcam image or the analyzed image with overlay to a PNG file on the USB flash drive connected to myRIO."
        n60 = call <vilib>:"Check if File or Folder Exists.vi"("error in (no error)"=w538, "path"=path "u:/") -> ("error out"=w537:errorcluster, "file or folder exists?"=w536:bool)  [unwired: 7 in, 1 out]
        n61 = case shown="True" w536 {
          tunnel: w543 -> [_ w556]
          tunnel: w540 -> [_ w555]
          tunnel: [w544 w554] -> w539
          tunnel: w537 -> [w544 w552]
          frame False {
            n62 = One Button Dialog(message="Please connect a USB flash drive\nto receive the image (use a USB hub)") -> ()  [unwired: 1 in, 1 out]
          }
          frame True {
            # "Save the currently-displayed image to disk"
            n63 = Unbundle By Name(w556) -> ("qsm.Analyzed image ref"=w551:T2, "qsm.Webcam image ref"=w557:T2)
            n64 = Unbundle By Name(w555) -> ("show analyzed"=w553:bool)
            n65 = Select(t=w551, s=w553, f=w557) -> (s? t:f=w550:T2)
            n66 = call "IMAQ Merge Overlay"("error in (no error)"=w552, "Image Src"=w550) -> ("error out"=w558:errorcluster, "Image Dst Out"=w549:T2)  [unwired: 8 in]
            n67 = Build Path(base path=path "u:/", name or relative path="image.png") -> (appended path=w547:path)
            n68 = call-poly "IMAQ Write File 2"("error in (no error)"=w558, "File Path"=w547, "Image"=w549) -> ("error out"=w554:errorcluster)  [unwired: 7 in, 1 out]
          }
        }
        n69 = Bundle By Name(cluster=w543, "save image"=FALSE) -> (w542:T4)
      }
      frame "state A" {
        w560 = FALSE
        w561 = TRUE
        # "Expansion State A"
        n70 = xnode "LED 3"("LED0"=w561, "LED1"=w560, "LED2"=w561, "LED3"=w560, "error in (no error)"=w562) -> ("error out"=w559:errorcluster)
      }
      frame "state B" {
        w607 = TRUE ("LED1")
        w608 = FALSE ("LED0")
        # "Expansion State B"
        n71 = xnode "LED 4"("LED0"=w608, "LED1"=w607, "LED2"=w608, "LED3"=w607, "error in (no error)"=w605) -> ("error out"=w606:errorcluster)
        n72 = Bundle By Name(cluster=w604, "save image"=FALSE) -> (w602:T4)
      }
      frame "state C" {
        # "Expansion State C"
        n73 = Unbundle By Name(w648) -> ("number img"=→"number img":i32)
      }
      frame "state D" {
        # "Expansion State D"
      }
      frame "state E" {
        # "Expansion State E"
      }
      frame "state F" {
        # "Expansion State F"
      }
      frame "state G" {
        # "Expansion State G"
      }
      frame "state H" {
        # "Expansion State H"
      }
    }
    n74 = case shown="\"two\"" "Enum" {
      tunnel: w22 -> [w88 _ w97 w107]
      frame "null", Default {
        n75 = Less Or Equal?(x=w88, y=650) -> (x <= y?=w86:bool)
        n76 = case shown="True" w86 {
          selector: w86 -> [_ w92]
          frame False {
            n77 = flat-sequence {
              frame #0 {
                n78 = local write "take"(FALSE ("take")) -> ()
              }
              frame #1 {
                n79 = local write "Reset Counter"(TRUE ("Reset Counter")) -> ()
              }
              frame #2 {
                n80 = local write "Reset Counter"(FALSE ("Reset Counter")) -> ()
              }
            }
          }
          frame True {
            n81 = flat-sequence {
              tunnel: w92 -> [w94]
              frame #0 {
                n82 = local write "Reset Counter"(FALSE) -> ()
              }
              frame #1 {
                n83 = local write "take"(w94) -> ()
              }
            }
          }
        }
      }
      frame "stop" {
        n84 = flat-sequence {
          frame #0 {
            n85 = local write "Reset Counter"(TRUE) -> ()
          }
        }
      }
      frame "one" {
        n86 = Less Or Equal?(x=w97, y=214) -> (x <= y?=w96:bool)
        n87 = case shown="True" w96 {
          selector: w96 -> [_ w102]
          frame False {
            n88 = flat-sequence {
              frame #0 {
                n89 = local write "take"(FALSE) -> ()
              }
              frame #1 {
                n90 = local write "Reset Counter"(TRUE) -> ()
              }
              frame #2 {
                n91 = local write "Reset Counter"(FALSE) -> ()
              }
            }
          }
          frame True {
            n92 = flat-sequence {
              tunnel: w102 -> [w104]
              frame #0 {
                n93 = local write "Reset Counter"(FALSE) -> ()
              }
              frame #1 {
                n94 = local write "take"(w104) -> ()
              }
            }
          }
        }
      }
      frame "two" {
        n95 = Less Or Equal?(x=w107, y=300) -> (x <= y?=w105:bool)
        n96 = case shown="True" w105 {
          selector: w105 -> [_ w111]
          frame False {
            n97 = flat-sequence {
              frame #0 {
                n98 = local write "take"(FALSE ("take")) -> ()
              }
              frame #1 {
                n99 = local write "Reset Counter"(TRUE ("Reset Counter")) -> ()
              }
              frame #2 {
                n100 = local write "Reset Counter"(FALSE ("Reset Counter")) -> ()
              }
            }
          }
          frame True {
            n101 = flat-sequence {
              tunnel: w111 -> [w113]
              frame #0 {
                n102 = local write "Reset Counter"(FALSE) -> ()
              }
              frame #1 {
                n103 = local write "take"(w113) -> ()
              }
            }
          }
        }
      }
    }
    n104 = Merge Errors(w23) -> (w13:errorcluster)
    n105 = local read "Num of Matches (Color Pattern Matching 1)"() -> (w8:i32)
    n106 = Greater?(x=w8, y=500) -> (0:w6:bool)
    n107 = case shown="True" w6 {
      frame False {
      }
      frame True {
        n108 = local read "Class (Particle Classification 1)"() -> (w48:string)
        n109 = local read "Classes (Color Classification 1)"() -> (w49:string[])
        n110 = Index Array(array=w49, index=1) -> (element=w47:string)
        n111 = Equal?(x=w48, y=w47) -> (x = y?=→"Pattern matches ball":bool)
      }
    }
    n112 = Merge Errors(w45, w13) -> (w14:errorcluster)
    "error out" <- w14
    n113 = call <vilib>:"Simple Error Handler.vi"() -> ()  [unwired: 5 in, 5 out]
  }
